vi "Set_Sorb_Power.vi"(8 "VISA session":refnum<visa-resource-name>="GPIB0::17::INSTR", 9 "Sorb Heater Resistance (Ohm)":dbl, 10 "Sorb Power (mW)":dbl, 11 "Sorb heater":bool) -> ()   [LabVIEW 2016]
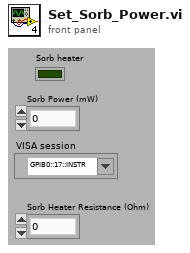
[diagram p1: front panel]
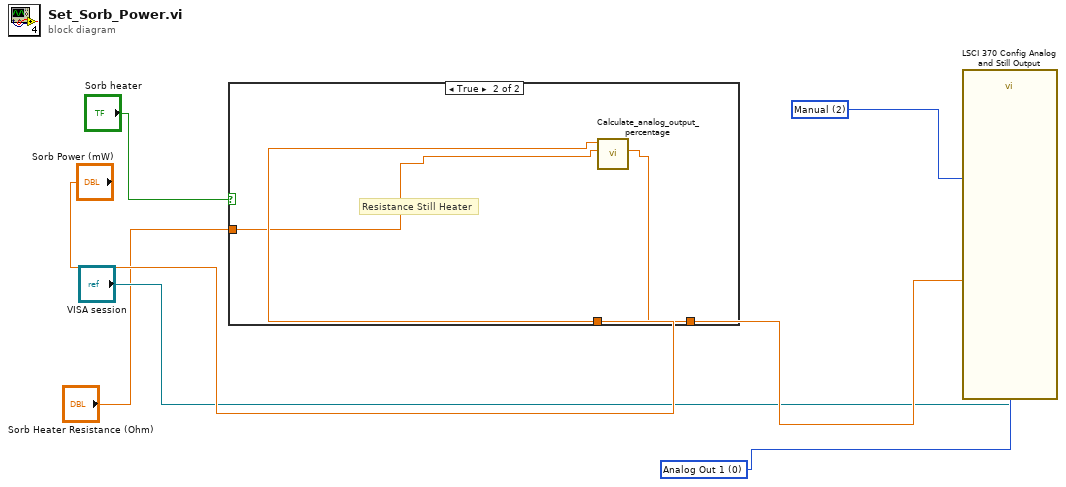
[diagram p0: block diagram]
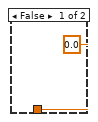
[diagram p2: hidden frame]
diagram:
  w6 = u16 0 items=["Analog Out 1", "Analog Out 2"] ("Analog Channel (0: Analog Out 1)")
  w7 = u16 2 items=["Off", "Channel", "Manual", "Zone", "Still"] ("Analog Out Mode (0: Off)")
  n1 = case shown="True" "Sorb heater" {
    tunnel: "Sorb Power (mW)" -> [_ w11]
    tunnel: [0.0 w10] -> w5
    tunnel: "Sorb Heater Resistance (Ohm)" -> [_ w9]
    frame False {
    }
    frame True {
      # "Resistance Still Heater"
      n2 = call "Calculate_analog_output_percentage.vi"("Resistance (Ohms)"=w9, "Power (mW)"=w11) -> ("Analog Output (%)"=w10:dbl)  [unwired: 9 in]
    }
  }
  n3 = call "LSCI 370 Config Analog and Still Output.vi"("VISA session"="VISA session", "Analog Out Mode (0: Off)"=w7, "Analog Channel (0: Analog Out 1)"=w6, "Manual Value (0.000)"=w5) -> ()  [unwired: 10 in, 2 out]
